vi "ingest.v2.vi"(6 "Properties and Labels":T1, 7 "Timestamp Metadata":refnum<class "timestampMetadata.lvclass">, 8 "error in":errorcluster, 9 "Title and Description":cluster{"Title":string, "Description":string}, 10 "S3 Path to File":string, 11 "Nominal Client in":refnum<class "Nominal Client.lvclass">) -> (0 "error out":errorcluster, 1 "Information":T2, 2 "datasetRid":string, 3 "Nominal Client out":refnum<class "Nominal Client.lvclass">, 4 "Response":string)   [LabVIEW 2020, in "Nominal Client.lvclass"]
doc: "Triggers an ingest job, allowing either creating a new dataset or uploading to an existing one. This endpoint is meant to supersede all other ingestion endpoints as their functionality gets migrated to this one."
uses:
  Nominal Client.lvclass
  timestampMetadata/timestampMetadata.lvclass
  4b965f09-dc68-4d5e-a5c1-32d476accfd4.vi
  3b653ec0-b3f4-4e20-9ef1-15560b52d02f.vi
  dc60078f-5e64-4343-b872-0272d4308f69.vi
  <vilib>/JDP Science/JSONtext/Variant to JSON Text.vi
  <vilib>/JDP Science/JSONtext/Array of Variants to JSON Object.vi
  <vilib>/JDP Science/JSONtext/Set Item.vi
  <vilib>/JDP Science/JSONtext/JSON text to Variant.vi
  <vilib>/JDP Science/JSONtext/LVClass Serializer/JSONtext LVClass Serializer.lvclass
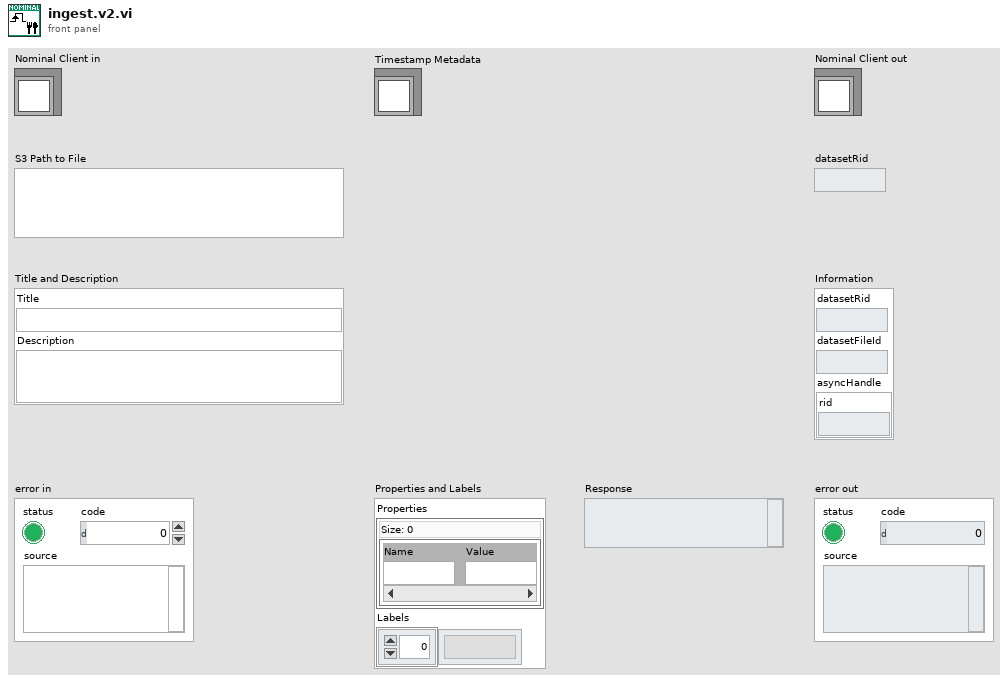
[diagram p1: front panel]
types:
  T1 = cluster{"Properties":map{string, string}, "Labels":string[]}
  T2 = cluster{"datasetRid":string, "datasetFileId":string, "asyncHandle":cluster{"rid":string}}
  T3 = cluster{"type":string, "s3":cluster{"path":string}}
  T4 = cluster{"source":cluster{"type":string, "s3":cluster{"path":string}}, "properties":string, "labels":string[], "datasetName":string, "datasetDescription":string}
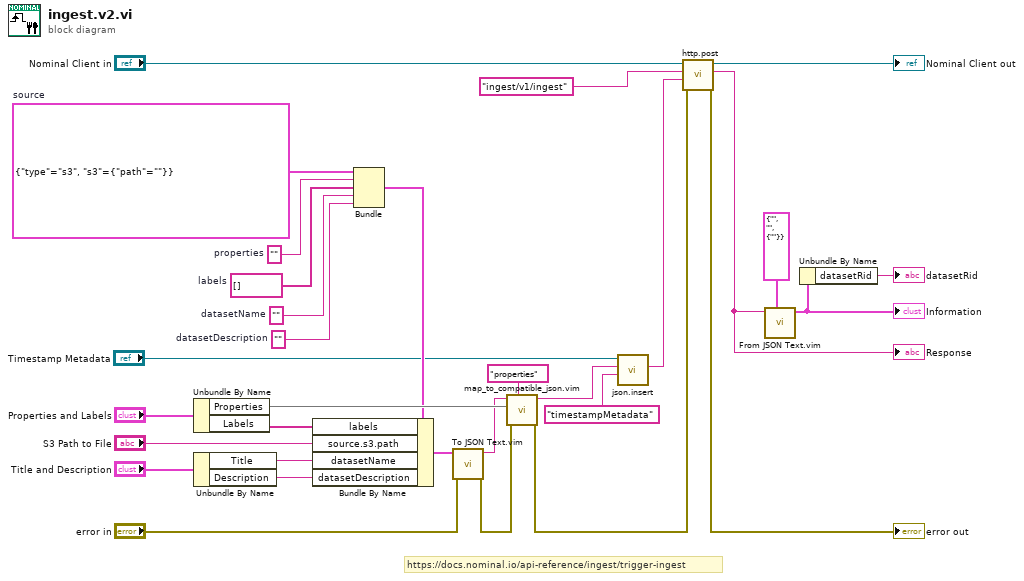
[diagram p0: block diagram]
diagram:
  w22 = ""  # datasetDescription
  w23 = ""  # datasetName
  w25 = ""  # properties
  w24 = string[] []  # labels
  w27 = T3 {"type"="s3", "s3"={"path"=""}}  # source
  # "https://docs.nominal.io/api-reference/ingest/trigger-ingest"
  n1 = Unbundle By Name("Properties and Labels") -> ("Properties"=w15:map{string, string}, "Labels"=w16:string[])
  n2 = Unbundle By Name("Title and Description") -> ("Title"=w18:string, "Description"=w19:string)
  n3 = Bundle("source"=w27, "properties"=w25, "labels"=w24, "datasetName"=w23, "datasetDescription"=w22) -> (w9:T4)  [unwired: 1 in]
  n4 = Bundle By Name(cluster=w9, "labels"=w16, "source.s3.path"="S3 Path to File", "datasetName"=w18, "datasetDescription"=w19) -> (w7:T4)
  n5 = call "To JSON Text.vim"("error in (no error)"="error in", "Anything"=w7) -> ("error out"=w5:errorcluster, "<JSON>"=w6:string)  [unwired: 8 in]
  n6 = call "map_to_compatible_json.vim"("JSON Path"="properties" ("Data Name"), "error in"=w5, "Map"=w15, "JSON in"=w6) -> ("error out"=w13:errorcluster, "JSON out"=w3:string)  [unwired: 6 in]
  n7 = call "json.insert.vi"("Object Name"="timestampMetadata", "JSON in"=w3, "timestampMetadata in"="Timestamp Metadata") -> ("JSON out"=w2:string)  [unwired: 6 in, 2 out]
  n8 = call "http.post.vi"("error in"=w13, "Request body"=w2, "Path"="ingest/v1/ingest", "Nominal Client in"="Nominal Client in") -> ("error out"=→"error out":errorcluster, "Response"=w10:string, "Nominal Client out"=→"Nominal Client out":refnum<class "Nominal Client.lvclass">)  [unwired: 4 in, 1 out]
  "Response" <- w10
  n9 = call "From JSON Text.vim"("Data Type and Default Value"=T2 {"datasetRid"="", "datasetFileId"="", "asyncHandle"={"rid"=""}} ("Information"), "JSON"=w10) -> ("Data out"=w12:T2)  [unwired: 8 in, 1 out]
  "Information" <- w12
  n10 = Unbundle By Name(w12) -> ("datasetRid"=→"datasetRid":string)
